vi "Write Image.vi"(8 "error in (no error)":errorcluster, 9 "Paths":path[](array[path]), 10 "ImageWriteBuffer":u16[](array[numeric]), 11 "ImageHandler in":refnum<class "ImageHandler.lvclass">) -> (0 "error out":errorcluster, 3 "ImageHandler out":refnum<class "ImageHandler.lvclass">)   [LabVIEW 2021, in "ImageHandler.lvlib" / "ImageHandler.lvclass"]
uses:
  ImageHandler.lvclass
  C:/Program Files/National Instruments/LabVIEW 2021/vi.lib/ActorFramework/Actor/Actor.lvclass
  ImageHandler.lvclass/ImageHandler.ctl
  <vilib>/ActorFramework/Actor/Actor.lvclass/Actor.ctl
  ImageHandler - Controller -- Interface/ImageHandler - Controller -- Interface Messages/Acquisition Status Msg/Acquisition Status Msg.lvclass/Acquisition Status Msg.ctl
  <vilib>/ActorFramework/Message Enqueuer/Message Enqueuer.lvclass/Message Enqueuer.ctl
  <vilib>/ActorFramework/Message Enqueuer/Enqueue.vi
  ImageHandler - Controller -- Interface/ImageHandler - Controller -- Interface Messages/Acquisition Status Msg/Acquisition Status Msg.lvclass
  C:/Program Files/National Instruments/LabVIEW 2021/vi.lib/ActorFramework/Message/Message.lvclass
  <vilib>/ActorFramework/Message Priority Queue/Priority Enqueue.vi
  <vilib>/ActorFramework/Actor/Actor.lvclass
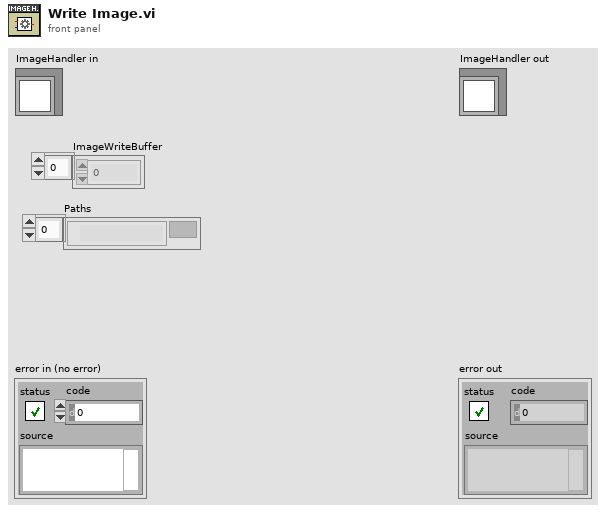
[diagram p1: front panel]
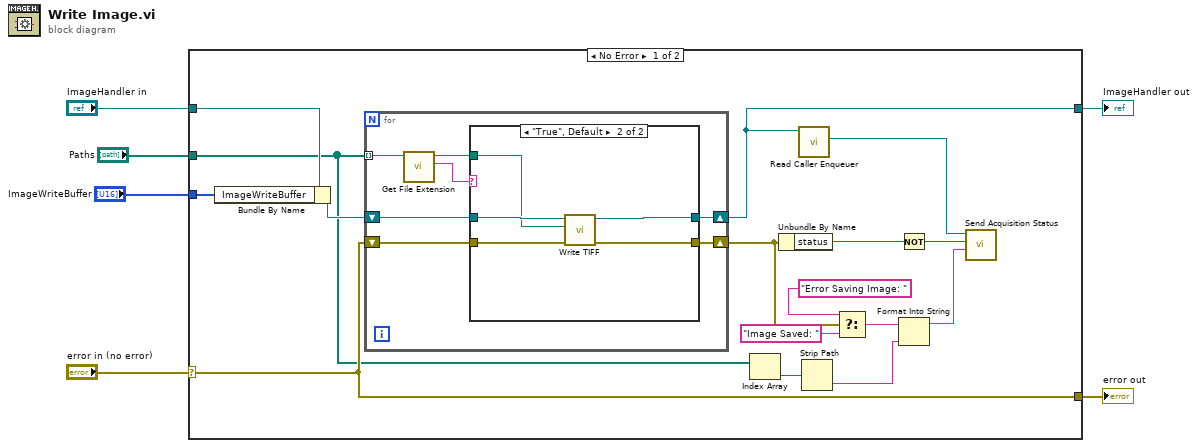
[diagram p0: block diagram]
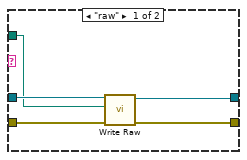
[diagram p2: hidden frame]
diagram:
  n1 = case shown="No Error" "error in (no error)" {
    selector: "error in (no error)" -> [w8 w41]
    tunnel: [w8 w41] -> w5
    tunnel: [w16 w40] -> w3
    tunnel: "ImageHandler in" -> [w18 w40]
    tunnel: "Paths" -> [w7 _]
    tunnel: "ImageWriteBuffer" -> [w17 _]
    frame No Error {
      n2 = Bundle By Name(cluster=w18, "ImageWriteBuffer"=w17) -> (w19:refnum<class "ImageHandler.lvclass">)
      n3 = for {
        tunnel: w7 -> [w25] mode=indexing
        shift-right: [w28] -> w13
        shift-left: w8 -> [w27]
        shift-right: [w29] -> w16
        shift-left: w19 -> [w26]
        n4 = call <vilib>:"Get File Extension.vi"("file"=w25) -> ("lowercase file extension"=w23:string, "dup file"=w24:path)  [unwired: 6 in, 3 out]
        n5 = case shown="\"True\", Default" w23 {
          tunnel: w26 -> [w34 w39]
          tunnel: [w33 w38] -> w29
          tunnel: w27 -> [w32 w37]
          tunnel: [w31 w36] -> w28
          tunnel: w24 -> [w30 w35]
          frame "raw" {
            n6 = call "Write Raw.vi"("error in (no error)"=w32, "Path"=w30, "ImageHandler in"=w34) -> ("error out"=w31:errorcluster, "ImageHandler out"=w33:refnum<class "ImageHandler.lvclass">)  [unwired: 7 in]
          }
          frame "True", Default {
            n7 = call "Write TIFF.vi"("error in (no error)"=w37, "Path"=w35, "ImageHandler in"=w39) -> ("error out"=w36:errorcluster, "ImageHandler out"=w38:refnum<class "ImageHandler.lvclass">)  [unwired: 7 in]
          }
        }
      }
      n8 = Index Array(array=w7) -> (element=w12:path)  [unwired: 1 in]
      n9 = Unbundle By Name(w13) -> ("status"=w21:bool)
      n10 = call <vilib>:"Read Caller Enqueuer.vi"("Actor"=w16) -> ("Caller Enqueuer"=w22:refnum<class "Message Enqueuer.lvclass">)  [unwired: 10 in]
      n11 = Strip Path(path=w12) -> (name=w11:string)  [unwired: 1 out]
      n12 = Select(t="Error Saving Image: ", s=w13, f="Image Saved: ") -> (s? t:f=w15:string)
      n13 = Not(x=w21) -> (.not. x?=w20:bool)
      n14 = Format Into String(initial string=w15, w11) -> (resulting string=w10:string)  [unwired: 2 in, 1 out]
      n15 = call "Send Acquisition Status.vi"("Remarks"=w10, "Status"=w20, "Message Enqueuer"=w22) -> ()  [unwired: 7 in, 2 out]
    }
    frame Error {
    }
  }
  "error out" <- w5
  "ImageHandler out" <- w3
